vi "Error 5001 - Error Reading JSON Message.vi"() -> (0 "error out":errorcluster)   [LabVIEW 2021]
doc: "Error 5001 - Error while reading JSON message. An empty string was read, or there was no '{' character in the string, or the string was malformed"
uses:
  <vilib>/Utility/error.llb/Error Cluster From Error Code.vi
  <vilib>/ErrorRing/Error Ring.xnode
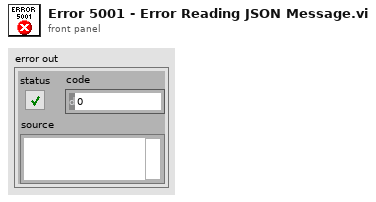
[diagram p1: front panel]
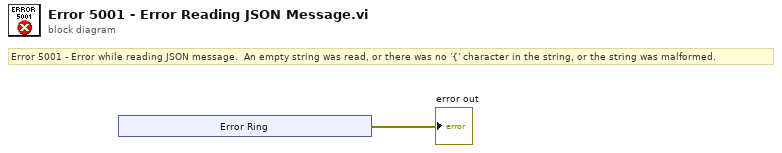
[diagram p0: block diagram]
diagram:
  # "Error 5001 - Error while reading JSON message.  An empty string was read, or there was no '{' character in the string, or the string was malformed."
  n1 = xnode "Error Ring"() -> ("error out"=→"error out":errorcluster)
